vi "sub extract RSSI phase and freq_demoinfocom.vi"(10 "multiple tone information":T1(array[cluster]), 11 "coerced IQ rate":dbl) -> (1 "Phase offset of both tones":dbl[](array[numeric]), 2 "RSSI of first tone 2":dbl, 3 "Frequency of first tone":dbl, 4 "Frequency list":dbl[](array[numeric]), 5 "Phase list":dbl[](array[numeric]))   [LabVIEW 2021]
uses:
  <vilib>/Analysis/coordinate.llb/Angle Range (Degree).ctl
  <vilib>/Analysis/coordinate.llb/Angle Units.ctl
  <vilib>/Analysis/coordinate.llb/Wrap Angle (scalar).vi
  <vilib>/Analysis/NI_AAL_Angle.lvlib
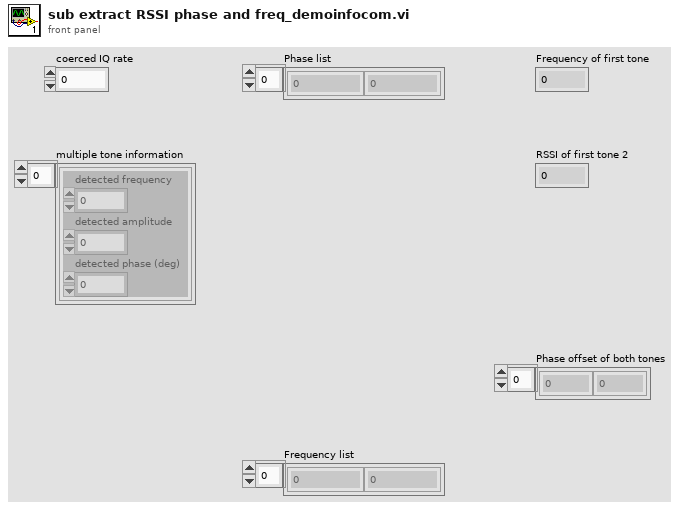
[diagram p1: front panel]
types:
  T1 = cluster{"detected frequency":dbl, "detected amplitude":dbl, "detected phase (deg)":dbl}[]
  T2 = typedef "NI_AAL_Angle.lvlib/Angle Units.ctl" = i32
  T3 = typedef "NI_AAL_Angle.lvlib/Angle Range (Degree).ctl" = u16
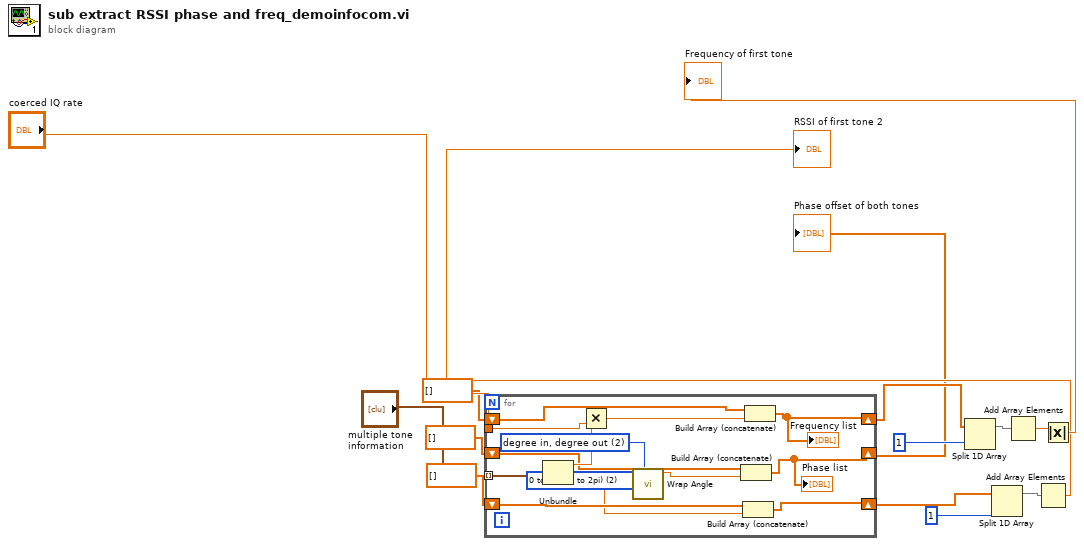
[diagram p0: block diagram]
diagram:
  n1 = for {
    tunnel: "multiple tone information" -> [w30] mode=indexing
    shift-right: [w28] -> w6
    shift-left: dbl[] [] -> [w29]
    tunnel: "coerced IQ rate" -> [w26]
    shift-right: [w25] -> w5
    shift-left: dbl[] [] -> [w21]
    shift-right: [w22] -> w13
    shift-left: dbl[] [] -> [w24]
    w16 = T2 2 items=["radian in, radian out", "radian in, degree out", "degree in, degree out", "degree in, radian out"] ("angle units")
    w18 = T3 2 items=["none", "-180 to 180 (-pi to pi)", "0 to 360 (0 to 2pi)"] ("angle range")
    n2 = Unbundle(w30) -> ("detected frequency"=w27:dbl, "detected amplitude"=w23:dbl, "detected phase (deg)"=w19:dbl)
    n3 = Multiply(x=w27, y=w26) -> (x*y=w20:dbl)
    n4 = call-poly <vilib>:"Wrap Angle.vi"("angle units"=w16, "angle range"=w18, "angle in"=w19) -> ("angle out"=w17:dbl)  [unwired: 7 in, 1 out]
    n5 = Build Array (concatenate)(w21, w17) -> (w25:dbl[])
    "Phase list" <- w25
    n6 = Build Array (concatenate)(w24, w23) -> (w22:dbl[])
    n7 = Build Array (concatenate)(w29, w20) -> (w28:dbl[])
    "Frequency list" <- w28
  }
  "Phase offset of both tones" <- w5
  n8 = Split 1D Array(array=w6, index=1) -> (first subarray=w8:dbl[])  [unwired: 1 out]
  n9 = Split 1D Array(array=w13, index=1) -> (first subarray=w12:dbl[])  [unwired: 1 out]
  n10 = Add Array Elements(numeric array=w8) -> (sum=w9:dbl)
  n11 = Add Array Elements(numeric array=w12) -> (sum=→"RSSI of first tone 2":dbl)
  n12 = Absolute Value(x=w9) -> (abs(x)=→"Frequency of first tone":dbl)
